vi "Get External Ignore List.vi"() -> (2 "Success?":bool, 3 "Lower case external ignores":string[](array[string]))   [LabVIEW 2019, in "Project.Dependencies Finder.lvlib"]
uses:
  Project.Dependencies Finder.lvlib
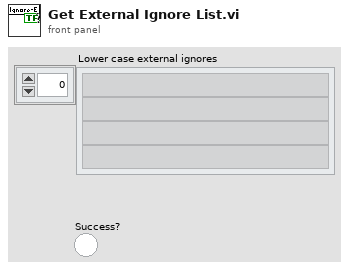
[diagram p1: front panel]
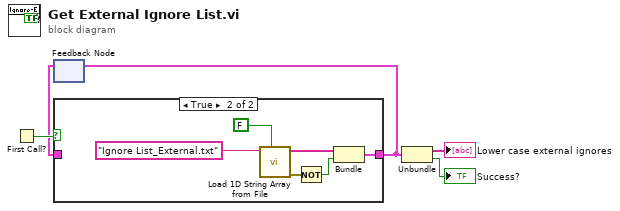
[diagram p0: block diagram]
diagram:
  n1 = First Call?() -> (First Call?: T/F=w5:bool)
  n2 = feedback #1() -> (w1:cluster{"Loaded 1D String Array":string[], bool})  [unwired: 1 in]
  n3 = case shown="True" w5 {
    tunnel: [w6 w11] -> w2
    tunnel: w1 -> [w6 _]
    frame False {
    }
    frame True {
      n4 = call "Load 1D String Array from File.vi"("Remove empty strings?(T)"=FALSE, "File name"="Ignore List_External.txt" ("name or relative path")) -> ("error out"=w8:errorcluster, "Loaded 1D String Array"=w9:string[])  [unwired: 8 in]
      n5 = Not(x=w8) -> (.not. x?=w12:bool)
      n6 = Bundle("Loaded 1D String Array"=w9, w12) -> (w11:cluster{"Loaded 1D String Array":string[], bool})  [unwired: 1 in]
    }
  }
  n7 = feedback-in #1(w2) -> ()
  n8 = Unbundle(w2) -> ("Loaded 1D String Array"=→"Lower case external ignores":string[], →"Success?":bool)
